vi "ValidateProjectPath.vi"(8 "error in (no error)":errorcluster, 11 "SetConditionalSymbol in":refnum<class "SetConditionalSymbol.lvclass">) -> (0 "error out":errorcluster, 3 "SetConditionalSymbol out":refnum<class "SetConditionalSymbol.lvclass">)   [LabVIEW 2014, in "SetConditionalSymbol.lvclass"]
uses:
  SetConditionalSymbol.lvclass
  SetConditionalSymbol.lvclass/SetConditionalSymbol.ctl
  <nishared>/LabVIEW CLI/Operations/Utilities/OperationErrorType.ctl
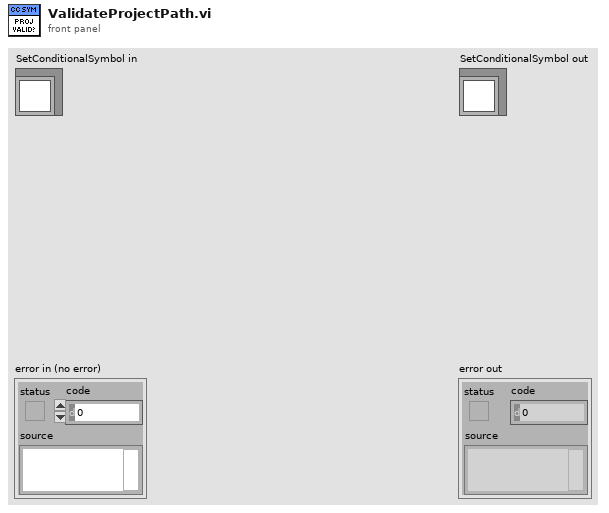
[diagram p1: front panel]
types:
  T1 = typedef "OperationErrorType.ctl" = enum16{"RequiredArgumentMissing", "UnknownArguments", "LoggerSetMultipleTimes", "OperationBrokenError"}
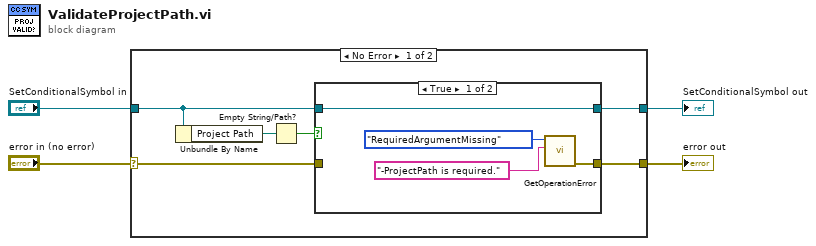
[diagram p0: block diagram]
diagram:
  n1 = case shown="No Error" "error in (no error)" {
    selector: "error in (no error)" -> [w9 w18]
    tunnel: [w5 w18] -> w3
    tunnel: [w8 w17] -> w1
    tunnel: "SetConditionalSymbol in" -> [w7 w17]
    frame No Error {
      n2 = Unbundle By Name(w7) -> ("Project Path"=w6:path)
      n3 = Empty String/Path?(string/path=w6) -> (empty?=w10:bool)
      n4 = case shown="True" w10 {
        tunnel: w9 -> [_ w16]
        tunnel: [w13 w16] -> w5
        tunnel: w7 -> [w14 w15]
        tunnel: [w14 w15] -> w8
        frame True {
          n5 = call <nishared>:"GetOperationError.vi"("Additional Information"="-ProjectPath is required.", "Operation Error Type"=OperationErrorType."RequiredArgumentMissing") -> ("error out"=w13:errorcluster)  [unwired: 9 in]
        }
        frame False {
        }
      }
    }
    frame Error {
    }
  }
  "error out" <- w3
  "SetConditionalSymbol out" <- w1
